vi "PhotonCamera_GetCameraMatrix.vi"(9 "BaseNTName":string="/photonvision", 11 "CameraName":string) -> (0 "error out":errorcluster, 3 "CameraMatrix":T1)   [LabVIEW 2019, in "PhotonVisionLib.lvlib"]
doc: "Returns the camera matrix\n\nInputs:\n - cameraName -- The nickname of the camera (found in the PhotonVision UI).\n \nOutputs:\n - CameraMatrix - matrix - 3 x 3 matrix of camera intrinsics. If empty, nothing was returned or nothing exists."
uses:
  PhotonVisionLib.lvlib
  <vilib>/Analysis/Matrix/Datatypes/RealMatrix.ctl
  <vilib>/Rock Robotics/WPI/ThirdParty/JAS_Junk/TrajLib/MatBuilder_Create.vi
  <vilib>/Rock Robotics/Network Tables/NT Read Numeric Array.vi
  <vilib>/Rock Robotics/WPI/ThirdParty/JAS_Junk/TrajLib/Trajectory_Library.lvlib
  <vilib>/Analysis/Matrix/NI_Matrix.lvlib
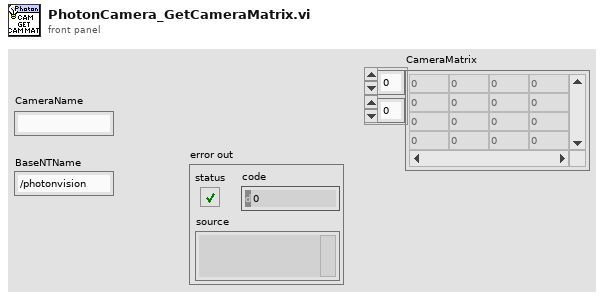
[diagram p1: front panel]
types:
  T1 = typedef "NI_Matrix.lvlib/RealMatrix.ctl" = dbl[][]
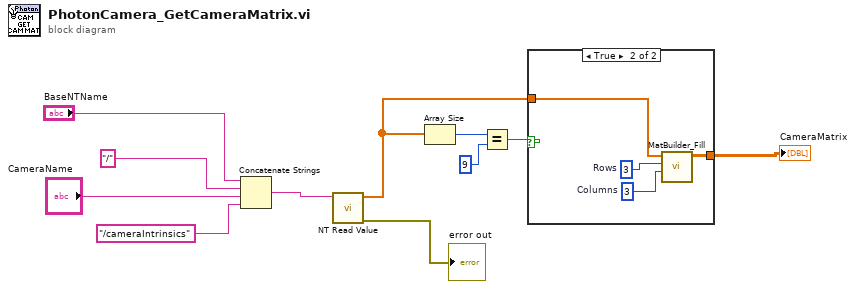
[diagram p0: block diagram]
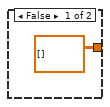
[diagram p2: hidden frame]
diagram:
  n1 = Concatenate Strings("BaseNTName", "/", "CameraName", "/cameraIntrinsics") -> (w8:string)
  n2 = call-poly <vilib>:"NT Read Value.vi"("name"=w8) -> ("error out"=→"error out":errorcluster, "value"=w3:dbl[])  [unwired: 8 in, 1 out]
  n3 = Array Size(array=w3) -> (size(s)=w6:i32)
  n4 = Equal?(x=w6, y=9) -> (x = y?=w4:bool)
  n5 = case shown="True" w4 {
    tunnel: w3 -> [_ w14]
    tunnel: [T1 [] ("output matrix") w13] -> w2
    frame False {
    }
    frame True {
      w16 = 3  # Columns
      w15 = 3  # Rows
      n6 = call <vilib>:"MatBuilder_Fill.vi"("Columns"=w16, "Rows"=w15, "Value List"=w14) -> ("output matrix"=w13:T1)  [unwired: 8 in]
    }
  }
  "CameraMatrix" <- w2
